vi "Comparison of LDA and PCA 2D projection.vi"() -> ()   [LabVIEW 2020]
doc: "The Iris dataset represents 3 kind of Iris flowers (Setosa, Versicolour and Virginica) with 4 attributes: sepal length, sepal width, petal length and petal width.\n\nPrincipal Component Analysis (PCA) applied to this data identifies the combination of attributes (principal components, or directions in the feature space) that account for the most variance in the data. Here we plot the different samples on the 2 first principal components.\n\nLinear Discriminant Analysis (LDA) tries to identify attributes that account for the most variance between classes. In particular, LDA, in contrast to PCA, is a supervised method, using known class labels."
uses:
  Model/Unsupervised/Decomposition/PCA/Controls/pca_params.ctl
  Model/Supervised/DiscriminantAnalysis/LinearDiscriminantAnalysis/Controls/linear_discriminant_analysis_params.ctl
  Display/Classification/2D/Predicted/Controls/PredictedParameter.ctl
  Display/_Controls/Style.ctl
  Model/Unsupervised/Decomposition/PCA/PCA.lvclass
  C:/Users/cipop/TDF Dropbox/2_Technologies de France/1 - Services et Etudes/PLAIY/2 - DEV/PLAIYLAB/code/Model/Model.lvclass
  Model/Supervised/DiscriminantAnalysis/LinearDiscriminantAnalysis/LinearDiscriminantAnalysis.lvclass
  C:/Users/cipop/TDF Dropbox/2_Technologies de France/1 - Services et Etudes/PLAIY/2 - DEV/PLAIYLAB/code/Model/Supervised/DiscriminantAnalysis/DiscriminantAnalysis.lvclass
  Model/Unsupervised/Decomposition/PCA/PCA.vi
  Model/Supervised/DiscriminantAnalysis/LinearDiscriminantAnalysis/LinearDiscriminantAnalysis.vi
panel:
  out "error out":errorcluster
  in  "error in":errorcluster
  in  "Local":T1
  out "Plot":cluster{"X":dbl[], "Y":dbl[]}[](graph) caption="PCA  of iris dataset"
  out "Plot 2":cluster{"X":dbl[], "Y":dbl[]}[](graph) caption="LDA of IRIS dataset"
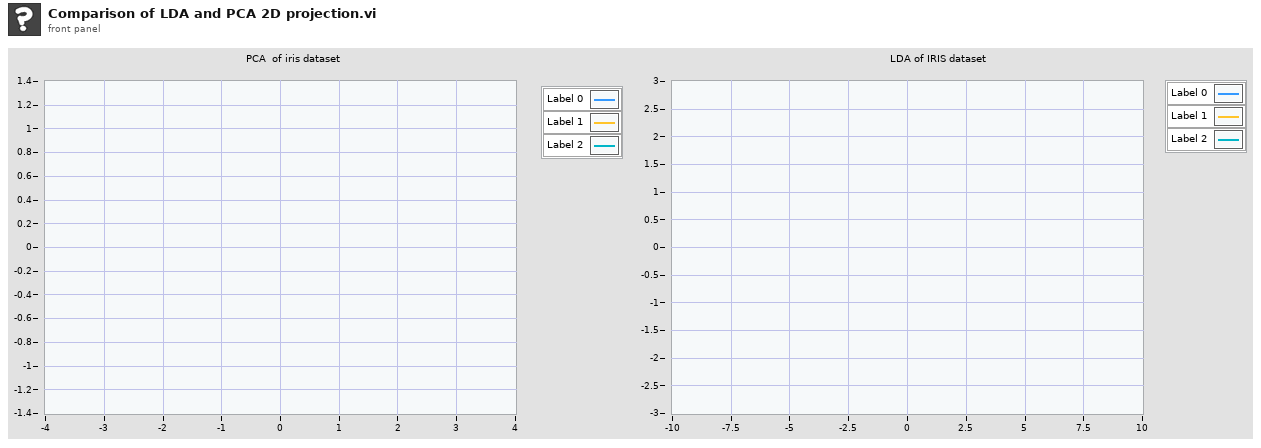
[diagram p1: front panel]
types:
  T1 = cluster{"X":dbl[][], "y":dbl[], "X_r":dbl[][], "X_r2":dbl[][]}
  T2 = typedef "pca_params.ctl" = cluster{"n_components":cluster{"n_components_type":string, "n_components_int":i32, "n_components_float":dbl}, "copy":bool, "whiten":bool, "svd_solver":string, "tol":dbl, "iterated_power":cluster{"iterated_power_type":string, "iterated_power_int":dbl}, "random_state":dbl}
  T3 = typedef "linear_discriminant_analysis_params.ctl" = cluster{"solver":string, "shrinkage":cluster{"shrinkage_type":string, "shrinkage_float":dbl}, "priors":cluster{"priors_type":string, "priors_list":dbl[]}, "n_components":cluster{"n_components_type":string, "n_components_int":dbl}, "store_covariance":bool, "tol":dbl}
  T4 = typedef "Style.ctl" = enum16{"Empty circle", "Full circle", "Empty square", "Full square", "Cross"}
  T5 = typedef "PredictedParameter.ctl" = cluster{"Plot":refnum<vi>, "Data":cluster{"X":dbl[][], "Predict":dbl[][]}, "Indexe":cluster{"X":i32, "Y":i32}, "Point Property":cluster{"Style":T4, "Label Color":u32[]}}
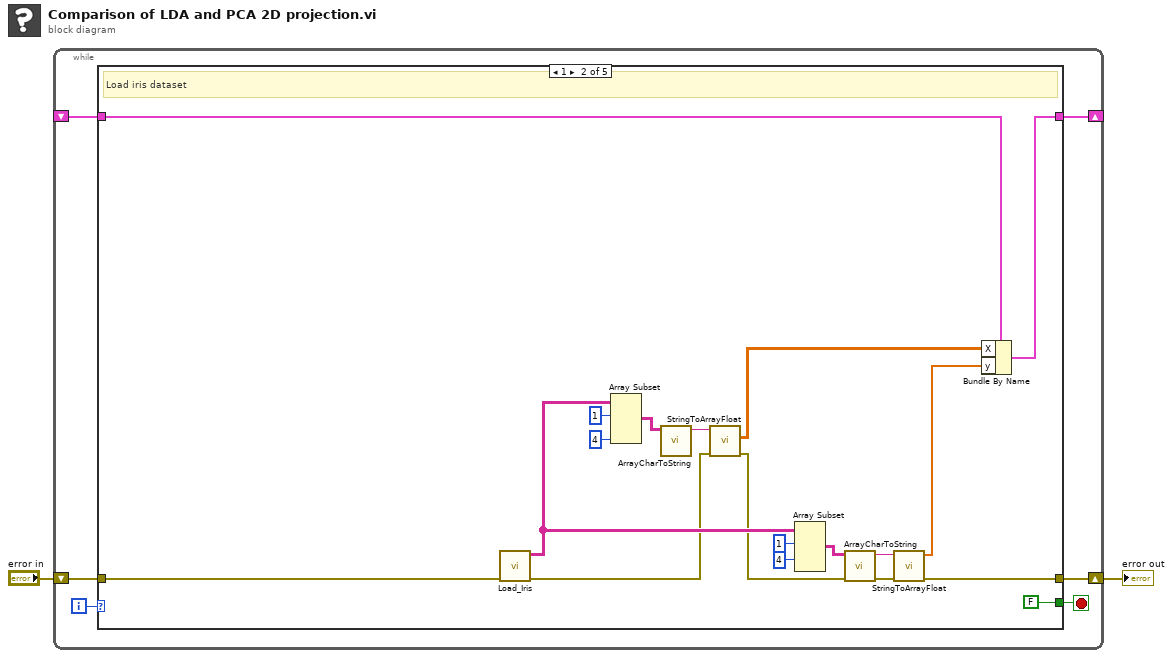
[diagram p0: block diagram]
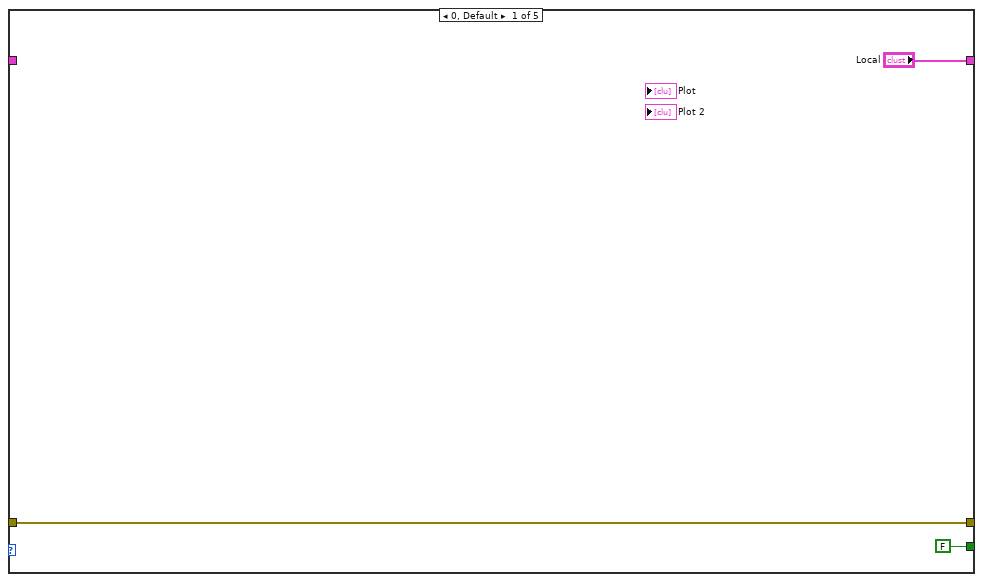
[diagram p2: hidden frame]
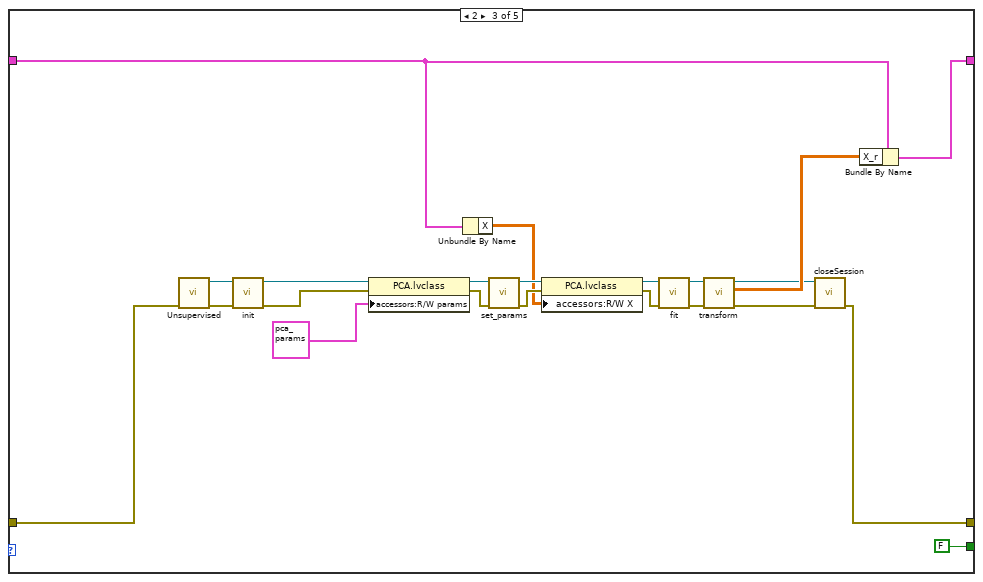
[diagram p3: hidden frame]
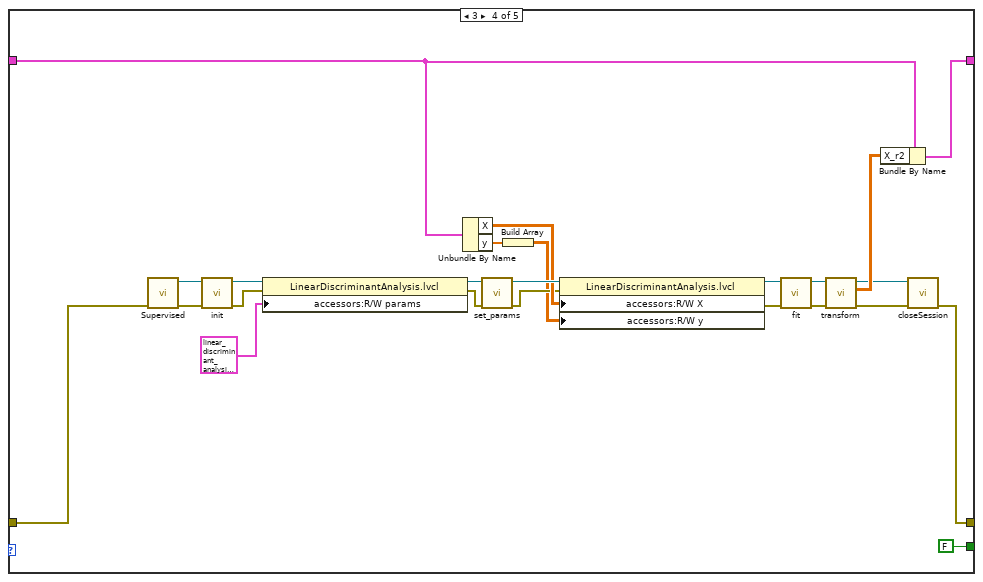
[diagram p4: hidden frame]
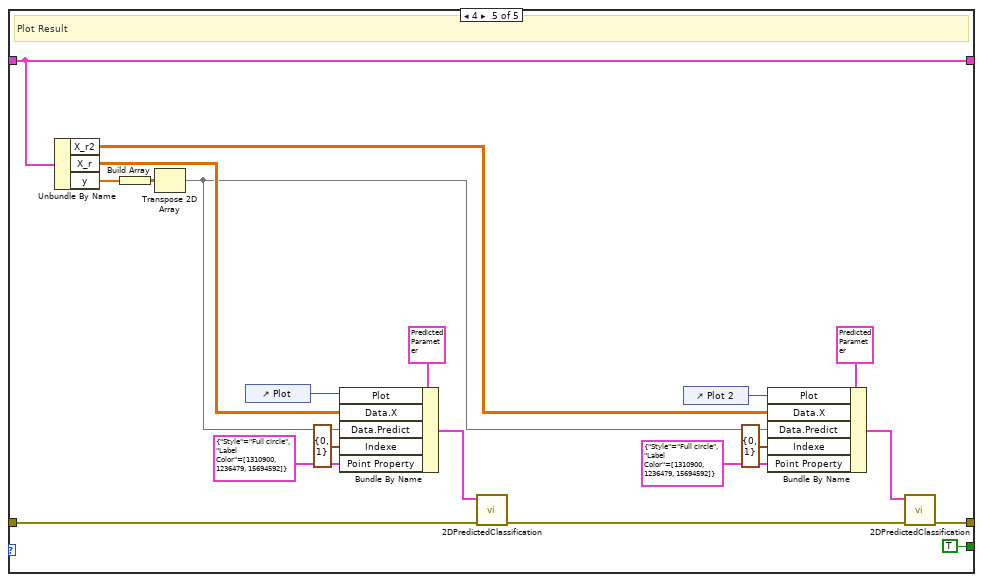
[diagram p5: hidden frame]
diagram:
  n1 = while {
    shift-right: [w6] -> w1
    shift-left: "error in" -> [w7]
    shift-right: [w5] -> _
    shift-left: _ -> [w4]
    i -> [w8]
    stop <- w3 stop-if-true
    n2 = case shown="1" w8 {
      tunnel: w7 -> [w10 w16 w40 w56 w92]
      tunnel: [w10 w13 w38 w67 w80] -> w6
      tunnel: ["Local" w27 w44 w69 w76] -> w5
      tunnel: w4 -> [_ w28 w45 w70 w76]
      tunnel: [FALSE FALSE FALSE FALSE TRUE] -> w3
      frame 0, Default {
      }
      frame 1 {
        # "Load iris dataset"
        n3 = call "Load_Iris.vi"("error in"=w16) -> ("error out"=w17:errorcluster, "Tableau"=w22:string[][])  [unwired: 9 in]
        n4 = Array Subset(array=w22, index (row)=1 ("index"), length (col)=4 ("length")) -> (w20:string[][])  [unwired: 2 in]
        n5 = call "ArrayCharToString.vi"("TAB"=w20) -> ("Instruction"=w21:string)  [unwired: 10 in]
        n6 = call "StringToArrayFloat.vi"("entrée d'erreur (pas d'erreur)"=w17, "Return value"=w21) -> ("error IO"=w14:errorcluster, "2DArray"=w15:dbl[][])  [unwired: 7 in, 1 out]
        n7 = Array Subset(array=w22, index (row)=1 ("index"), index (col)=4 ("index")) -> (w18:string[][])  [unwired: 2 in]
        n8 = call "ArrayCharToString.vi"("TAB"=w18) -> ("Instruction"=w19:string)  [unwired: 10 in]
        n9 = call "StringToArrayFloat.vi"("entrée d'erreur (pas d'erreur)"=w14, "Return value"=w19) -> ("error IO"=w13:errorcluster, "1DArray"=w12:dbl[])  [unwired: 7 in, 1 out]
        n10 = Bundle By Name(cluster=w28, "X"=w15, "y"=w12) -> (w27:T1)
      }
      frame 2 {
        n11 = call-poly "Unsupervised.vi"("error in"=w40) -> ("error out"=w41:errorcluster, "out"=w42:refnum<class "PCA.lvclass">)  [unwired: 9 in]
        n12 = call-dynamic "init.vi"("error in (no error)"=w41, "Model en entrée"=w42) -> ("error out"=w46:errorcluster, "Model en sortie"=w50:refnum<class "PCA.lvclass">)  [unwired: 8 in]
        n13 = property class="PCA.lvclass"(reference=w50, error in=w46, "accessors:R/W params"=T2 {"n_components"={"n_components_type"="int", "n_components_int"=2, "n_components_float"=0.0}, "copy"=TRUE, "whiten"=FALSE, "svd_solver"="auto", "tol"=0.0, "iterated_power"={"iterated_power_type"="auto", "iterated_power_int"=0.0}, "random_state"=0.0} ("R/W params")) -> (reference out=w49:refnum<class "PCA.lvclass">, error out=w43:errorcluster)
        n14 = Unbundle By Name(w45) -> ("X"=w39:dbl[][])
        n15 = call-dynamic "set_params.vi"("error in (no error)"=w43, "PCA.lvclass 2"=w49) -> ("error out"=w47:errorcluster, "PCA.lvclass"=w48:refnum<class "PCA.lvclass">)  [unwired: 8 in]
        n16 = property class="PCA.lvclass"(reference=w48, error in=w47, "accessors:R/W X"=w39) -> (reference out=w37:refnum<class "PCA.lvclass">, error out=w36:errorcluster)
        n17 = call-dynamic "fit.vi"("error in (no error)"=w36, "Decomposition.lvclass 2"=w37) -> ("error out"=w30:errorcluster, "Decomposition.lvclass"=w31:refnum<class "PCA.lvclass">)  [unwired: 8 in]
        n18 = call-dynamic "transform.vi"("error in (no error)"=w30, "Decomposition.lvclass 2"=w31) -> ("error out"=w33:errorcluster, "X_new"=w35:dbl[][], "Decomposition.lvclass"=w34:refnum<class "PCA.lvclass">)  [unwired: 7 in]
        n19 = call-dynamic "closeSession.vi"("error in"=w33, "Python en entrée"=w34) -> ("error out"=w38:errorcluster)  [unwired: 8 in, 1 out]
        n20 = Bundle By Name(cluster=w45, "X_r"=w35) -> (w44:T1)
      }
      frame 3 {
        n21 = call-poly "Supervised.vi"("error in"=w56) -> ("error out"=w57:errorcluster, "out"=w58:refnum<class "LinearDiscriminantAnalysis.lvclass">)  [unwired: 9 in]
        n22 = call-dynamic "init.vi"("error in (no error)"=w57, "Model en entrée"=w58) -> ("error out"=w71:errorcluster, "Model en sortie"=w74:refnum<class "LinearDiscriminantAnalysis.lvclass">)  [unwired: 8 in]
        n23 = property class="LinearDiscriminantAnalysis.lvcl"(reference=w74, error in=w71, "accessors:R/W params"=T3 {"solver"="svd", "shrinkage"={"shrinkage_type"="None", "shrinkage_float"=0.0}, "priors"={"priors_type"="None", "priors_list"=[]}, "n_components"={"n_components_type"="int", "n_components_int"=2.0}, "store_covariance"=FALSE, "tol"=0.0001} ("R/W params")) -> (reference out=w73:refnum<class "LinearDiscriminantAnalysis.lvclass">, error out=w55:errorcluster)
        n24 = Unbundle By Name(w70) -> ("X"=w68:dbl[][], "y"=w53:dbl[])
        n25 = call-dynamic "set_params.vi"("error in (no error)"=w55, "LinearDiscriminantAnalysis.lvclass 2"=w73) -> ("error out"=w54:errorcluster, "LinearDiscriminantAnalysis.lvclass"=w72:refnum<class "LinearDiscriminantAnalysis.lvclass">)  [unwired: 8 in]
        n26 = Build Array(w53) -> (w52:dbl[][])
        n27 = property class="LinearDiscriminantAnalysis.lvcl"(reference=w72, error in=w54, "accessors:R/W X"=w68, "accessors:R/W y"=w52) -> (reference out=w66:refnum<class "LinearDiscriminantAnalysis.lvclass">, error out=w65:errorcluster)
        n28 = call-dynamic "fit.vi"("error in (no error)"=w65, "DiscriminantAnalysis.lvclass 2"=w66) -> ("error out"=w63:errorcluster, "DiscriminantAnalysis.lvclass"=w64:refnum<class "LinearDiscriminantAnalysis.lvclass">)  [unwired: 8 in]
        n29 = call-dynamic "transform.vi"("error in (no error)"=w63, "LinearDiscriminantAnalysis.lvclass 2"=w64) -> ("error out"=w60:errorcluster, "X_new"=w62:dbl[][], "LinearDiscriminantAnalysis.lvclass"=w61:refnum<class "LinearDiscriminantAnalysis.lvclass">)  [unwired: 7 in]
        n30 = Bundle By Name(cluster=w70, "X_r2"=w62) -> (w69:T1)
        n31 = call-dynamic "closeSession.vi"("error in"=w60, "Python en entrée"=w61) -> ("error out"=w67:errorcluster)  [unwired: 8 in, 1 out]
      }
      frame 4 {
        # "Plot Result"
        n32 = Unbundle By Name(w76) -> ("X_r2"=w78:dbl[][], "X_r"=w88:dbl[][], "y"=w90:dbl[])
        n33 = Build Array(w90) -> (w89:dbl[][])
        n34 = Transpose 2D Array(2D array=w89) -> (transposed array=w79:dbl[][])
        n35 = control-ref of="Plot"() -> (w91:refnum<vi>)
        n36 = Bundle By Name(cluster=T5 {"Plot"=refnum, "Data"={"X"=[], "Predict"=[]}, "Indexe"={"X"=0, "Y"=1}, "Point Property"={"Style"=enum."Full circle", "Label Color"=[8978528, 4367871, 1985280]}} ("Parameters"), "Plot"=w91, "Data.X"=w88, "Data.Predict"=w79, "Indexe"=cluster{"X":i32, "Y":i32} {"X"=0, "Y"=1}, "Point Property"=cluster{"Style":T4, "Label Color":u32[]} {"Style"=enum."Full circle", "Label Color"=[1310900, 1236479, 15694592]}) -> (w95:T5)
        n37 = call "2DPredictedClassification.vi"("error in"=w92, "Parameters"=w95) -> ("error out"=w81:errorcluster)  [unwired: 9 in]
        n38 = control-ref of="Plot 2"() -> (w77:refnum<vi>)
        n39 = Bundle By Name(cluster=T5 {"Plot"=refnum, "Data"={"X"=[], "Predict"=[]}, "Indexe"={"X"=0, "Y"=1}, "Point Property"={"Style"=enum."Full circle", "Label Color"=[8978528, 4367871, 1985280]}} ("Parameters"), "Plot"=w77, "Data.X"=w78, "Data.Predict"=w79, "Indexe"=cluster{"X":i32, "Y":i32} {"X"=0, "Y"=1}, "Point Property"=cluster{"Style":T4, "Label Color":u32[]} {"Style"=enum."Full circle", "Label Color"=[1310900, 1236479, 15694592]}) -> (w82:T5)
        n40 = call "2DPredictedClassification.vi"("error in"=w81, "Parameters"=w82) -> ("error out"=w80:errorcluster)  [unwired: 9 in]
      }
    }
  }
  "error out" <- w1
